vi "Polymerize 2.vi"(11 "Puzzle In":T1) -> (3 "Puzzle":T1)   [LabVIEW 2020]
uses:
  Puzzle 14-2.ctl
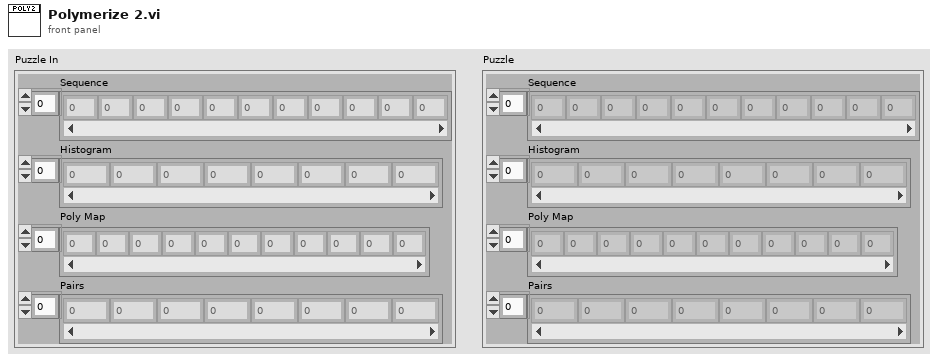
[diagram p1: front panel]
types:
  T1 = typedef "Puzzle 14-2.ctl" = cluster{"Sequence":u8[], "Histogram":i64[], "Poly Map":u8[], "Pairs":i64[]}
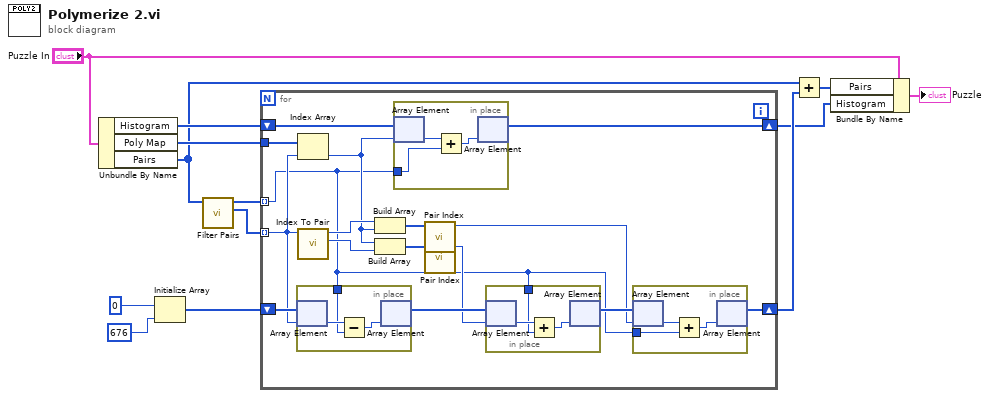
[diagram p0: block diagram]
diagram:
  n1 = Unbundle By Name("Puzzle In") -> ("Histogram"=w10:i64[], "Poly Map"=w11:u8[], "Pairs"=w3:i64[])
  n2 = Initialize Array(i64 0 ("element"), 676 ("dimension size")) -> (w9:i64[])
  n3 = call "Filter Pairs.vi"("Pairs"=w3) -> ("Array 2"=w1:i32[], "Array"=w2:i64[])  [unwired: 9 in]
  n4 = for {
    tunnel: w11 -> [w29]
    shift-right: [w27] -> w5
    shift-left: w10 -> [w28]
    shift-right: [w25] -> w8
    shift-left: w9 -> [w26]
    tunnel: w1 -> [w15] mode=indexing
    tunnel: w2 -> [w14] mode=indexing
    n5 = in-place {
      in-place-border: w14 -> [w36]
      n6 = in-place-array #1(w26, w15) -> (w38:i64)
      n7 = Subtract(x=w38, y=w36) -> (x-y=w37:i64)
      n8 = in-place-array #1(w37) -> (w19:i64[])  [unwired: 1 out]
    }
    n9 = Index Array(array=w29, index=w15) -> (element=w22:u8)
    n10 = call "Index To Pair.vi"("Index"=w15) -> ("Second"=w24:u8, "First"=w23:u8)  [unwired: 9 in]
    n11 = Build Array(w23, w22) -> (w21:u8[])
    n12 = Build Array(w22, w24) -> (w20:u8[])
    n13 = in-place {
      in-place-border: w14 -> [w40]
      n14 = in-place-array #2(w28, w22) -> (w41:i64)
      n15 = Add(x=w41, y=w40) -> (x+y=w39:i64)
      n16 = in-place-array #2(w39) -> (w27:i64[])  [unwired: 1 out]
    }
    n17 = call "Pair Index.vi"("Pair"=w21) -> ("Index"=w16:i32)  [unwired: 10 in]
    n18 = call "Pair Index.vi"("Pair"=w20) -> ("Index"=w18:i32)  [unwired: 10 in]
    n19 = in-place {
      in-place-border: w14 -> [w33]
      n20 = in-place-array #3(w19, w18) -> (w35:i64)
      n21 = Add(x=w35, y=w33) -> (x+y=w34:i64)
      n22 = in-place-array #3(w34) -> (w17:i64[])  [unwired: 1 out]
    }
    n23 = in-place {
      in-place-border: w14 -> [w30]
      n24 = in-place-array #4(w17, w16) -> (w32:i64)
      n25 = Add(x=w32, y=w30) -> (x+y=w31:i64)
      n26 = in-place-array #4(w31) -> (w25:i64[])  [unwired: 1 out]
    }
  }
  n27 = Add(x=w3, y=w8) -> (x+y=w6:i64[])
  n28 = Bundle By Name(cluster="Puzzle In", "Pairs"=w6, "Histogram"=w5) -> (→"Puzzle":T1)
